vi "Acquisition Message Loop.vi"(8 "error in (no error)":errorcluster, 9 "Data Queue":refnum<queue>, 10 "Data Notifiers":T1, 11 "Message Queues":T2) -> (0 "error out":errorcluster)   [LabVIEW 2013, in "Acquisition.lvlib"]
doc: "Message loop for handling messages pertaining to the acquisition of data from the hardware."
uses:
  Acquisition.lvlib
  support/Message Queue/All Message Queues.ctl
  support/Message Queue/Message Cluster.ctl
  support/Data Notifiers/All Data Notifiers.ctl
  APD Notifier Cluster.ctl
  Piezo/Piezo display.ctl
  XY/XY Display.ctl
  Capacitive/Capacitive Signal Cluster.ctl
  Acquisition State.ctl
  Hardware Configuration.ctl
  Counter Configuration.ctl
  ADC/ADC Configuration.ctl
  support/Message Queue/Enqueue Message (Single).vi
  <vilib>/Utility/error.llb/Error Cluster From Error Code.vi
  <vilib>/ErrorRing/Error Ring.xnode
  support/Message Queue/Message Queue.lvlib
  Piezo/Piezo.lvlib
  XY/XY.lvlib
  support/Data Notifiers/Data Notifiers.lvlib
  Capacitive/Capacitive.lvlib
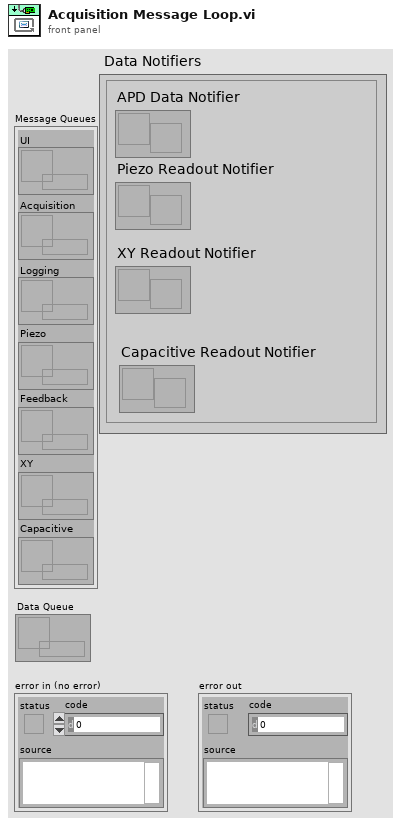
[diagram p1: front panel]
types:
  T1 = typedef "Data Notifiers.lvlib/All Data Notifiers.ctl" = cluster{"APD Data Notifier":refnum<notifier>, "Piezo Readout Notifier":refnum<notifier>, "XY Readout Notifier":refnum<notifier>, "Capacitive Readout Notifier":refnum<notifier>}
  T2 = typedef "Message Queue.lvlib/All Message Queues.ctl" = cluster{"UI":refnum<queue>, "Acquisition":refnum<queue>, "Logging":refnum<queue>, "Piezo":refnum<queue>, "Feedback":refnum<queue>, "XY":refnum<queue>, "Capacitive":refnum<queue>}
  T3 = typedef "Acquisition.lvlib/Hardware Configuration.ctl" = cluster{"Data Source":u16, "Counter Configuration":T4, "ADC Configuration":T5}
  T4 = typedef "Acquisition.lvlib/Counter Configuration.ctl" = cluster{"DAQmx Task":refnum<k21>, "Counter(s)":tag, "samples per readout":i32}
  T5 = typedef "Acquisition.lvlib/ADC Configuration.ctl" = cluster{"DAQmx Task":refnum<k21>, "Channel(s)":tag, "samples per readout":i32, "Sample Rate (s/s)":i32, "Max Voltage":dbl, "Min Voltage":dbl}
  T6 = typedef "Acquisition.lvlib/Acquisition State.ctl" = enum16{"Idle", "Acquiring"}
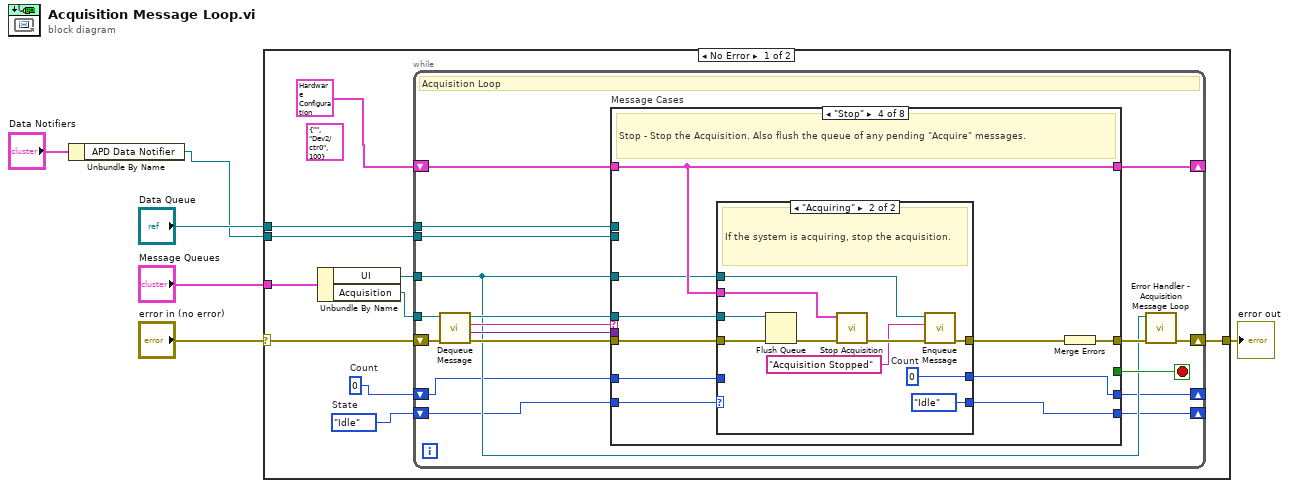
[diagram p0: block diagram]
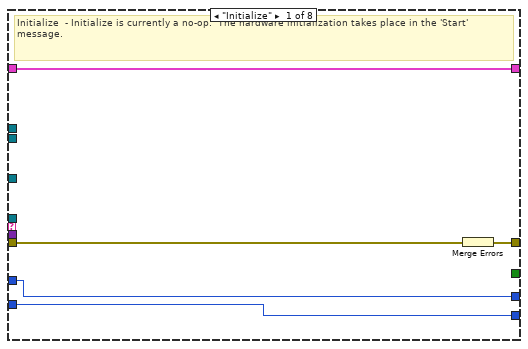
[diagram p2: hidden frame]
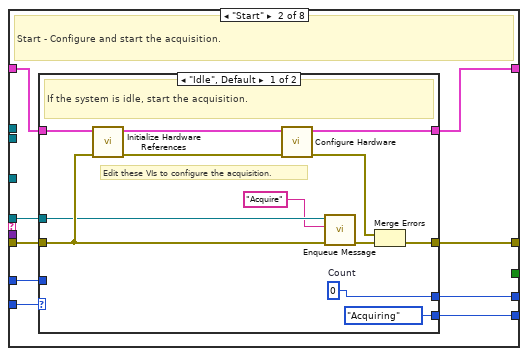
[diagram p3: hidden frame]
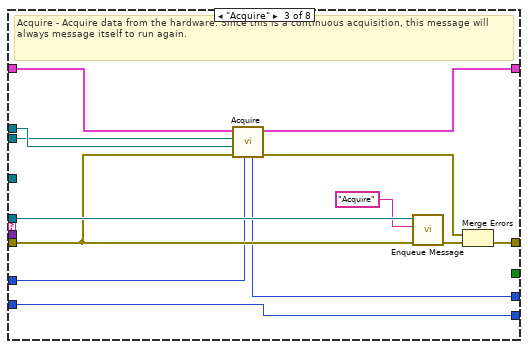
[diagram p5: hidden frame]
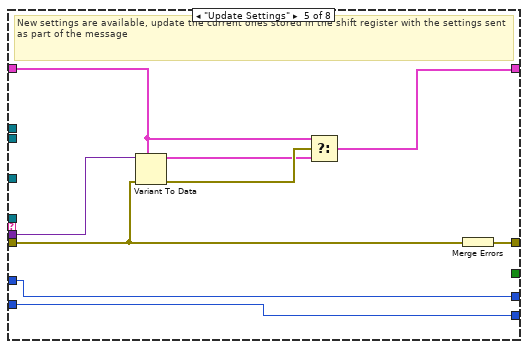
[diagram p7: hidden frame]
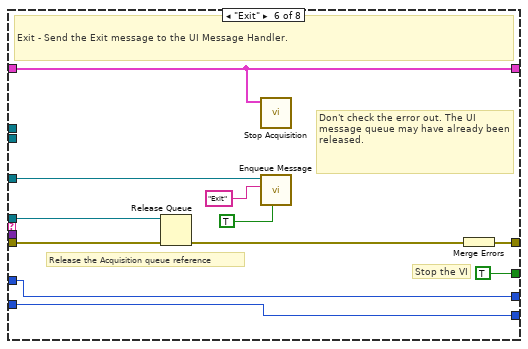
[diagram p8: hidden frame]
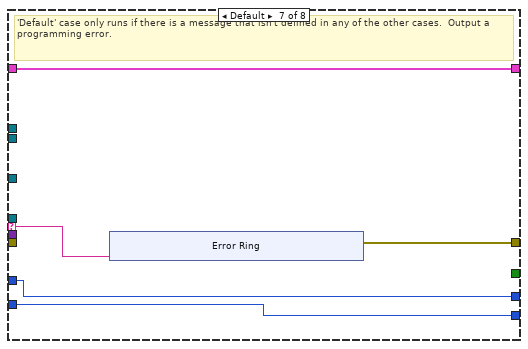
[diagram p9: hidden frame]
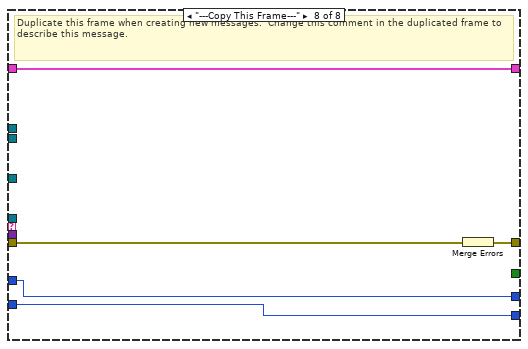
[diagram p10: hidden frame]
diagram:
  n1 = Unbundle By Name("Data Notifiers") -> ("APD Data Notifier"=w1:refnum<notifier>)
  n2 = case shown="No Error" "error in (no error)" {
    selector: "error in (no error)" -> [w13 w138]
    tunnel: "Message Queues" -> [w16 _]
    tunnel: [w14 w138] -> w5
    tunnel: "Data Queue" -> [w11 _]
    tunnel: w1 -> [w9 _]
    frame No Error {
      (unwired) T4 {"DAQmx Task"="", "Counter(s)"="Dev2/ctr0", "samples per readout"=100} ("Counter Configuration")
      w8 = 0  # Count
      w10 = Acquisition_State."Idle"  # State
      n3 = Unbundle By Name(w16) -> ("UI"=w12:refnum<queue>, "Acquisition"=w15:refnum<queue>)
      n4 = while {
        tunnel: w15 -> [w26]
        shift-right: [w33] -> _
        shift-left: T3 {"Data Source"=0, "Counter Configuration"={"DAQmx Task"="", "Counter(s)"="Dev2/ctr0", "samples per readout"=100}, "ADC Configuration"={"DAQmx Task"="", "Channel(s)"="Dev2/ctr0", "samples per readout"=100, "Sample Rate (s/s)"=0, "Max Voltage"=0.0, "Min Voltage"=0.0}} ("Acquisition Config") -> [w34]
        shift-right: [w23] -> w14
        shift-left: w13 -> [w31]
        tunnel: w12 -> [w22]
        tunnel: w11 -> [w25]
        shift-right: [w20] -> _
        shift-left: w10 -> [w21]
        tunnel: w9 -> [w19]
        shift-right: [w18] -> _
        shift-left: w8 -> [w17]
        stop <- w32 stop-if-true
        # "Acquisition Loop"
        n5 = call "Dequeue Message.vi"("error in (no error)"=w31, "Message Queue"=w26) -> ("error out"=w30:errorcluster, "Message Data"=w28:variant, "Message"=w29:string, "dup Message Queue"=w27:refnum<queue>)  [unwired: 6 in]
        n6 = case "Message Cases" shown="\"Stop\"" w29 {
          selector: w29 -> [_ _ _ _ _ _ w124 _]
          tunnel: w27 -> [_ w45 w75 w84 _ w113 _ _]
          tunnel: w30 -> [w38 w46 w74 w86 w103 w117 _ w137]
          tunnel: [w39 w48 w77 w87 w109 w119 w123 w135] -> w24
          tunnel: w34 -> [w37 w47 w71 w85 w105 w112 w125 w136]
          tunnel: [w37 w44 w72 w85 w104 w112 w125 w136] -> w33
          tunnel: [_ _ _ _ _ TRUE _ _] -> w32
          tunnel: w28 -> [_ _ _ _ w108 _ _ _]
          tunnel: w22 -> [_ _ _ w83 _ w118 _ _]
          tunnel: w25 -> [_ _ w69 _ _ _ _ _]
          tunnel: w21 -> [w36 w43 w68 w82 w102 w111 w122 w134]
          tunnel: [w36 w42 w68 w81 w102 w111 w122 w134] -> w20
          tunnel: w19 -> [_ _ w67 _ _ _ _ _]
          tunnel: [w35 w41 w65 w79 w101 w110 w121 w133] -> w18
          tunnel: w17 -> [w35 w40 w66 w78 w101 w110 w121 w133]
          frame "Initialize" {
            # "Initialize  - Initialize is currently a no-op.  The hardware initialization takes place in the 'Start' message."
            n7 = Merge Errors(w38) -> (w39:errorcluster)
          }
          frame "Start" {
            # "Start - Configure and start the acquisition."
            n8 = case shown="\"Idle\", Default" w43 {
              selector: w43 -> [_ w62]
              tunnel: [w60 w64] -> w48
              tunnel: w47 -> [w49 w63]
              tunnel: w46 -> [w59 w64]
              tunnel: w45 -> [w57 _]
              tunnel: [w53 w63] -> w44
              tunnel: [Acquisition_State."Acquiring" ("State") w62] -> w42
              tunnel: [w50 w61] -> w41
              tunnel: w40 -> [_ w61]
              frame "Idle", Default {
                w50 = 0  # Count
                # "Edit these VIs to configure the acquisition."
                # "If the system is idle, start the acquisition."
                n9 = call "Initialize Hardware References.vi"("error in (no error)"=w59, "HW Resources In"=w49) -> ("error out"=w56:errorcluster, "HW Resources Out"=w54:T3)  [unwired: 8 in]
                n10 = call "Configure Hardware.vi"("error in (no error)"=w56, "HW Resources In"=w54) -> ("error out"=w55:errorcluster, "HW Resources Out"=w53:T3)  [unwired: 8 in]
                n11 = call-poly "Enqueue Message.vi"("error in (no error)"=w59, "Message"="Acquire", "Message Queue"=w57) -> ("error out"=w58:errorcluster)  [unwired: 7 in, 1 out]
                n12 = Merge Errors(w55, w58) -> (w60:errorcluster)
              }
              frame "Acquiring" {
                # "The system is already acquiring. Ignore the \"Start\" message."
              }
            }
          }
          frame "Acquire" {
            # "Acquire - Acquire data from the hardware. Since this is a continuous acquisition, this message will always message itself to run again."
            n13 = call "Acquire.vi"("Count In"=w66, "error in (no error)"=w74, "Data Queue"=w69, "Data Notifier"=w67, "HW Resources In"=w71) -> ("error out"=w73:errorcluster, "HW Resources Out"=w72:T3, "Cout Out"=w65:i32)  [unwired: 4 in]
            n14 = call-poly "Enqueue Message.vi"("error in (no error)"=w74, "Message"="Acquire", "Message Queue"=w75) -> ("error out"=w76:errorcluster)  [unwired: 7 in, 1 out]
            n15 = Merge Errors(w73, w76) -> (w77:errorcluster)
          }
          frame "Stop" {
            # "Stop - Stop the Acquisition. Also flush the queue of any pending \"Acquire\" messages."
            n16 = case shown="\"Acquiring\"" w82 {
              selector: w82 -> [w90 _]
              tunnel: w86 -> [w89 w100]
              tunnel: w85 -> [_ w99]
              tunnel: w84 -> [_ w97]
              tunnel: w83 -> [_ w96]
              tunnel: [w90 Acquisition_State."Idle" ("State")] -> w81
              tunnel: [w89 w94] -> w80
              tunnel: [w88 w91] -> w79
              tunnel: w78 -> [w88 _]
              frame "Idle", Default {
                # "The system is already idle. Ignore the \"Stop\" message."
              }
              frame "Acquiring" {
                w91 = 0  # Count
                # "If the system is acquiring, stop the acquisition."
                n17 = Flush Queue(queue=w97, error in (no error)=w100) -> (error out=w98:errorcluster)  [unwired: 2 out]
                n18 = call "Stop Acquisition.vi"("error in (no error)"=w98, "HW Resources In"=w99) -> ("error out"=w95:errorcluster)  [unwired: 9 in]
                n19 = call-poly "Enqueue Message.vi"("error in (no error)"=w95, "Message"="Acquisition Stopped", "Message Queue"=w96) -> ("error out"=w94:errorcluster)  [unwired: 7 in, 1 out]
              }
            }
            n20 = Merge Errors(w80) -> (w87:errorcluster)
          }
          frame "Update Settings" {
            # "New settings are available, update the current ones stored in the shift register with the settings sent as part of the message"
            n21 = Variant To Data(error in=w103, type=w105, Variant=w108) -> (data=w106:T3, error out=w107:errorcluster)
            n22 = Select(t=w105, s=w107, f=w106) -> (s? t:f=w104:T3)
            n23 = Merge Errors(w103) -> (w109:errorcluster)
          }
          frame "Exit" {
            # "Don't check the error out. The UI message queue may have already been released."
            # "Release the Acquisition queue reference"
            # "Stop the VI"
            # "Exit - Send the Exit message to the UI Message Handler."
            n24 = Release Queue(queue=w113, error in (no error)=w117) -> (error out=w114:errorcluster)  [unwired: 1 in, 2 out]
            n25 = call "Stop Acquisition.vi"("HW Resources In"=w112) -> ()  [unwired: 10 in, 1 out]
            n26 = call-poly "Enqueue Message.vi"("Priority Message? (F)"=TRUE, "Message"="Exit", "Message Queue"=w118) -> ()  [unwired: 7 in, 2 out]
            n27 = Merge Errors(w114) -> (w119:errorcluster)
          }
          frame Default {
            # "'Default' case only runs if there is a message that isn't defined in any of the other cases.  Output a programming error."
            n28 = xnode "Error Ring"("parameter 0"=w124) -> ("error out"=w123:errorcluster)
          }
          frame "---Copy This Frame---" {
            # "Duplicate this frame when creating new messages.  Change this comment in the duplicated frame to describe this message."
            n29 = Merge Errors(w137) -> (w135:errorcluster)
          }
        }
        n30 = call "Error Handler - Acquisition Message Loop.vi"("error in (no error)"=w24, "Message Queue"=w22) -> ("dup error in"=w23:errorcluster)  [unwired: 8 in, 1 out]
      }
    }
    frame Error {
    }
  }
  "error out" <- w5
